vi "Read x (800).vi"(8 "error in (no error)":errorcluster, 11 "cosmetic changes in":refnum<class "cosmetic changes.lvclass">) -> (0 "error out":errorcluster, 2 "x (800)":i16=800, 3 "cosmetic changes out":refnum<class "cosmetic changes.lvclass">)   [LabVIEW 2013, in "cosmetic changes.lvclass"]
uses:
  cosmetic changes.lvclass
  cosmetic changes.lvclass/cosmetic changes.ctl
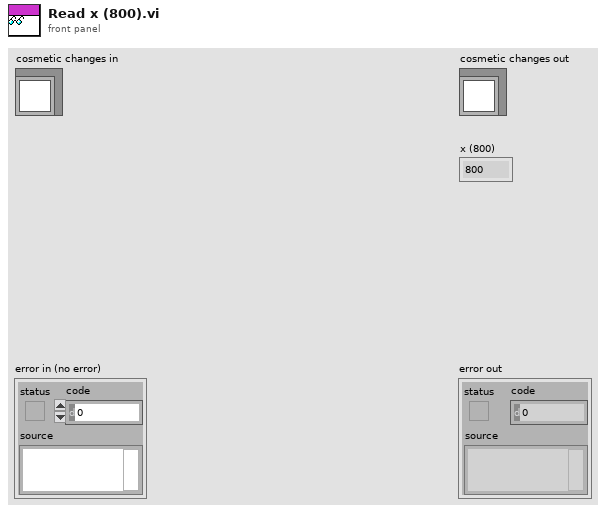
[diagram p1: front panel]
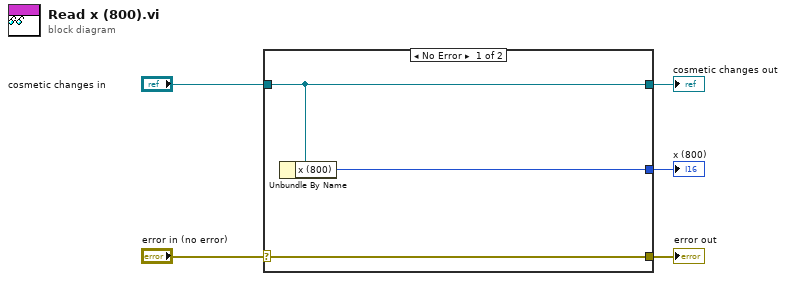
[diagram p0: block diagram]
diagram:
  n1 = case shown="No Error" "error in (no error)" {
    selector: "error in (no error)" -> [w8 w9]
    tunnel: [w8 w9] -> w4
    tunnel: [w7 w10] -> w2
    tunnel: "cosmetic changes in" -> [w7 w10]
    tunnel: [w6 _] -> w1
    frame No Error {
      n2 = Unbundle By Name(w7) -> ("x (800)"=w6:i16)
    }
    frame Error {
    }
  }
  "error out" <- w4
  "cosmetic changes out" <- w2
  "x (800)" <- w1
